vi "状态告警区.vi"(11 "数组":u16[](array[numeric]) format="%04xH") -> (3 "状态告警区":T1 {"工作状态" items=["空闲"=0, "水样测试"=1, "标样核查"=2, "零点核查"=3, "跨度核查"=4, "空白测试"=5, "平行样测试"=6, "加标回收"=7, "空白校准"=8, "标样校准"=9, "标定"=19, "初始化（清洗）"=10, "标样1测量"=28, "标样2测量"=29, "故障"=30, "异常处理"=31, "初始装液"=32, "其他"=33]; "告警代码" items=["无告警", "缺试剂告警", "缺水样告警", "缺蒸馏水告警", "缺标液告警", "仪表漏液告警", "标定异常告警", "超量程告警", "加热异常", "低试剂预警", "超上限告警", "超下限告警", "仪表内部其他异常", "滴定异常告警", "电极异常告警", "量程切换告警", "参数设置告警", "PH电极电位异常", "电导率电极异常", "浊度光度异常", "溶解氧电极异常", "溶解氧光强异常", "温度异常告警", "PH异常告警", "溶解氧异常告警", "电导率异常告警", "浊度异常告警", "叶绿素异常告警", "藻密度异常告警", "蓝绿藻异常告警", "ORP异常告警", "氨氮异常告警", "清洁刷异常告警", "SD卡异常告警", "蓝牙异常告警", "Wifi异常告警", "流程异常告警"]; "故障代码" items=["无故障", "电机故障", "温度故障", "通讯故障", "滴定故障"]})   [LabVIEW 2022 SP3, in "挥发酚.lvlib"]
panel:
  # "共占用10WORD"
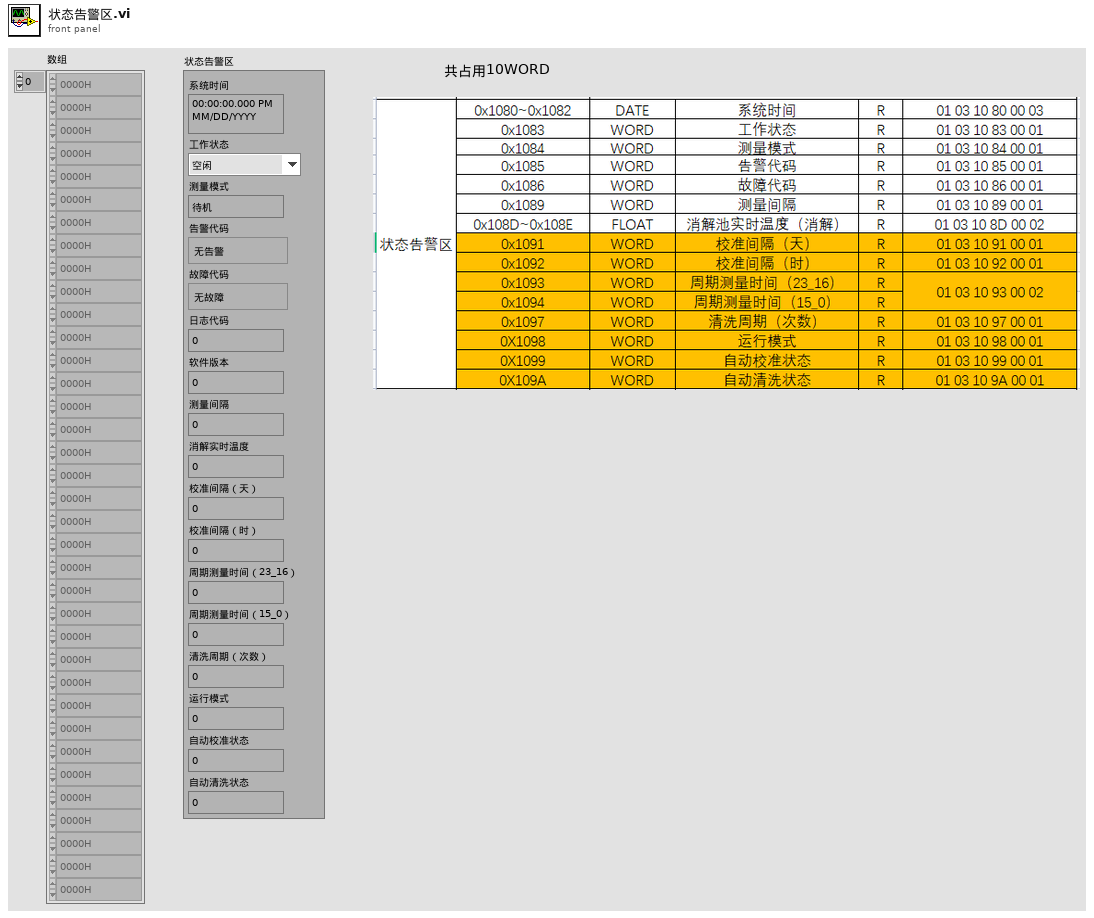
[diagram p1: front panel]
types:
  T1 = cluster{"系统时间":timestamp, "工作状态":u16, "测量模式":enum16{"待机", "连续模式", "周期模式", "定点模式", "受控模式", "手动模式"}, "告警代码":u16, "故障代码":u16, "日志代码":u16, "软件版本":u16, "测量间隔":u16, "消解实时温度":dbl, "校准间隔（天）":u16, "校准间隔（时）":u16, "周期测量时间（23_16）":u16, "周期测量时间（15_0）":u16, "清洗周期（次数）":u16, "运行模式":u16, "自动校准状态":u16, "自动清洗状态":u16}
  T2 = cluster{"time stamp":timestamp, "WORD":u16, "WORD":u16, "WORD":u16, "WORD":u16, "WORD":u16, "WORD":u16, "WORD":u16, "FLOAT":sgl, "WORD":u16, "WORD":u16, "WORD":u16, "WORD":u16, "WORD":u16, "WORD":u16, "WORD":u16, "WORD":u16}
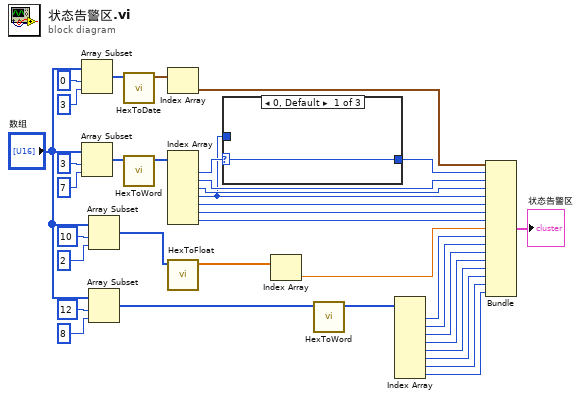
[diagram p0: block diagram]
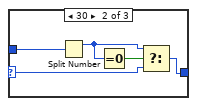
[diagram p2: hidden frame]
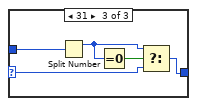
[diagram p3: hidden frame]
diagram:
  n1 = Array Subset(array="数组", index=0 ("索引"), length=3 ("长度")) -> (w34:u16[])
  n2 = Array Subset(array="数组", index=3 ("索引"), length=7 ("长度")) -> (w29:u16[])
  n3 = Array Subset(array="数组", index=10 ("索引"), length=2 ("长度")) -> (w22:u16[])
  n4 = Array Subset(array="数组", index=12 ("索引"), length=8 ("长度")) -> (w19:u16[])
  n5 = call "HexToDate.vi"("数组"=w34) -> ("DATE"=w31:timestamp[])  [unwired: 10 in]
  n6 = call "HexToWord.vi"("数组"=w29) -> ("WORD"=w28:u16[])  [unwired: 10 in]
  n7 = Index Array(array=w31) -> (element=w30:timestamp)  [unwired: 1 in]
  n8 = Index Array(array=w28) -> (element #1=w3:u16, element #2=w27:u16, element #3=w26:u16, element #4=w2:u16, element #5=w6:u16, element #6=w5:u16, element #7=w4:u16)  [unwired: 7 in]
  n9 = call "HexToFloat.vi"("数组"=w22) -> ("FLOAT"=w21:sgl[])  [unwired: 10 in]
  n10 = case shown="0, Default" w3 {
    selector: w3 -> [w37 w39 w43]
    tunnel: w2 -> [_ w42 w44]
    tunnel: [w37 w38 w45] -> w1
    frame 0, Default {
    }
    frame 30 {
      n11 = Split Number(x=w42) -> (hi(x)=w40:u8)  [unwired: 1 out]
      n12 = Equal To 0?(x=w40) -> (x = 0?=w41:bool)
      n13 = Select(t=w40, s=w41, f=w39) -> (s? t:f=w38:u16)
    }
    frame 31 {
      n14 = Split Number(x=w44) -> (hi(x)=w46:u8)  [unwired: 1 out]
      n15 = Equal To 0?(x=w46) -> (x = 0?=w47:bool)
      n16 = Select(t=w46, s=w47, f=w43) -> (s? t:f=w45:u16)
    }
  }
  n17 = Index Array(array=w21) -> (element=w20:sgl)  [unwired: 1 in]
  n18 = call "HexToWord.vi"("数组"=w19) -> ("WORD"=w15:u16[])  [unwired: 10 in]
  n19 = Index Array(array=w15) -> (element #1=w14:u16, element #2=w13:u16, element #3=w12:u16, element #4=w11:u16, element #5=w10:u16, element #6=w9:u16, element #7=w8:u16, element #8=w7:u16)  [unwired: 8 in]
  n20 = Bundle("time stamp"=w30, "WORD"=w1, "WORD"=w27, "WORD"=w26, "WORD"=w2, "WORD"=w6, "WORD"=w5, "WORD"=w4, "FLOAT"=w20, "WORD"=w14, "WORD"=w13, "WORD"=w12, "WORD"=w11, "WORD"=w10, "WORD"=w9, "WORD"=w8, "WORD"=w7) -> (→"状态告警区":T2)  [unwired: 1 in]
